vi "save_bin.vi"(2 "Signal":cluster{sgl, sgl, "Data Array":i16[][]}, 3 "timestamp":timestamp) -> ()   [LabVIEW 2010]
panel:
  out "appended path":path
  out "error out":errorcluster
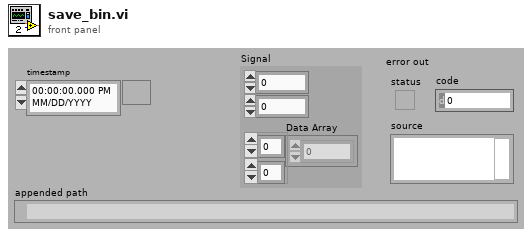
[diagram p1: front panel]
types:
  T1 = enum16{"deny read/write", "deny write-only", "deny none"}
  T2 = enum16{"open", "replace", "create", "open or create", "replace or create", "replace or create with confirmation"}
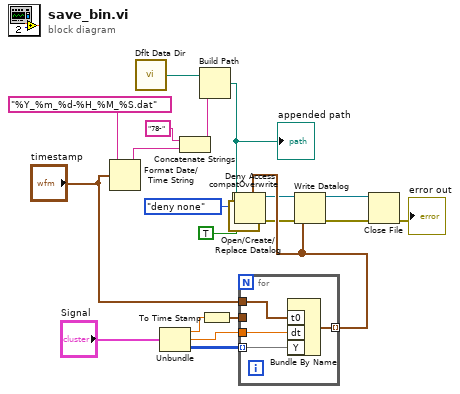
[diagram p0: block diagram]
diagram:
  n1 = Format Date/Time String(time format string (%c)="%Y_%m_%d-%H_%M_%S.dat", seconds (now)="timestamp") -> (date/time string=w17:string)  [unwired: 1 in]
  n2 = call <vilib>:"Dflt Data Dir.vi"() -> ("App:Default Data Directory"=w19:path)
  n3 = Unbundle("Signal") -> (w12:sgl, w13:sgl, "Data Array"=w14:i16[][])
  n4 = Concatenate Strings("78-" ("string"), w17) -> (w16:string)
  n5 = Build Path(base path=w19, name or relative path=w16) -> (appended path=w7:path)
  "appended path" <- w7
  n6 = To Time Stamp(1:w12) -> (0:w10:timestamp)
  n7 = call <vilib>:"compatOverwrite.vi"("overwrite (F)"=TRUE) -> ("overwrite?"=w1:T2)
  n8 = for {
    tunnel: w14 -> [w27] mode=indexing
    tunnel: w13 -> [w26]
    tunnel: w10 -> [_]
    tunnel: [w25] -> w9 mode=indexing
    tunnel: "timestamp" -> [w24]
    n9 = Bundle By Name("t0"=w24, "dt"=w26, "Y"=w27) -> (w25:waveform(i16))  [unwired: 1 in]
  }
  n10 = Open/Create/Replace Datalog(5:w9, 10:w1, 11:w7) -> (0:w3:errorcluster, 3:w2:refnum<k1>)  [unwired: 3 in, 1 out]
  n11 = Deny Access(4:w3, 6:T1."deny none" ("deny mode (2)"), 7:w2) -> (0:w6:errorcluster, 3:w8:refnum<k1>)
  n12 = Write Datalog(4:w6, 6:w9, 7:w8) -> (0:w21:errorcluster, 3:w22:refnum<k1>)
  n13 = Close File(refnum=w22, error in=w21) -> (error out=→"error out":errorcluster)  [unwired: 1 out]
